vi "copy excel template.vi"(8 "error in (no error)":errorcluster, 10 "report file path in":path, 11 "template file path in":path) -> (0 "error out":errorcluster, 1 "file  exists?":bool, 2 "report file path out":path)   [LabVIEW 2016]
uses:
  <vilib>/Utility/NIReport.llb/NI_report.lvclass
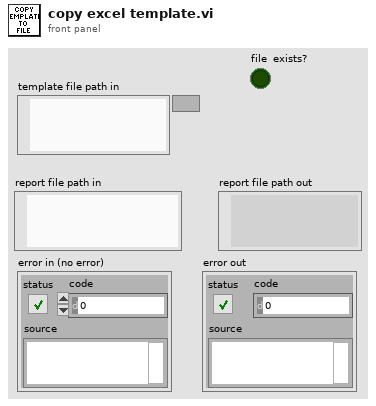
[diagram p1: front panel]
types:
  T1 = enum16{"maximized", "minimized", "normal", "no change"}
  T2 = enum16{"Standard Report", "HTML", "Word", "Excel"}
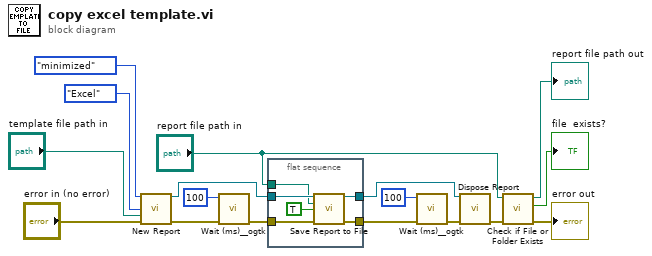
[diagram p0: block diagram]
diagram:
  n1 = call <vilib>:"New Report.vi"("window state (normal)"=T1."minimized", "report type"=T2."Excel", "template (empty)"="template file path in", "error in (no error)"="error in (no error)") -> ("report out"=w10:refnum<class "NI_report.lvclass">, "error out"=w12:errorcluster)  [unwired: 10 in]
  n2 = call <userlib>:"Wait (ms)__ogtk.vi"("error in (no error)"=w12, "milliseconds to wait"=u32 100) -> ("error out"=w9:errorcluster)  [unwired: 8 in, 1 out]
  n3 = flat-sequence {
    tunnel: [w23] -> w8
    tunnel: [w22] -> w7
    tunnel: w9 -> [w20]
    tunnel: w10 -> [w19]
    tunnel: "report file path in" -> [w18]
    frame #0 {
      n4 = call-dynamic "Save Report to File.vi"("report in"=w19, "report file path"=w18, "prompt to replace? (F)"=TRUE, "error in (no error)"=w20) -> ("report out"=w23:refnum<class "NI_report.lvclass">, "error out"=w22:errorcluster)  [unwired: 10 in]
    }
  }
  n5 = call <userlib>:"Wait (ms)__ogtk.vi"("error in (no error)"=w7, "milliseconds to wait"=u32 100) -> ("error out"=w6:errorcluster)  [unwired: 8 in, 1 out]
  n6 = call-dynamic "Dispose Report.vi"("report in"=w8, "error in (no error)"=w6) -> ("error out"=w17:errorcluster)  [unwired: 13 in]
  n7 = call <vilib>:"Check if File or Folder Exists.vi"("error in (no error)"=w17, "path"="report file path in") -> ("error out"=→"error out":errorcluster, "file or folder exists?"=→"file  exists?":bool, "dup path"=→"report file path out":path)  [unwired: 7 in]
